vi "Skm To Dkm.vi"(8 "error in (no error)":errorcluster, 10 "error":i32, 11 "sKilo":string) -> (0 "error out":i32, 1 "function return":dbl, 2 "error out 2":errorcluster, 3 "sKilo out":string)   [LabVIEW 2023, in "POSCONV.lvlib"]
doc: "double SkmToDkm(char *sKilo, int *error);"
uses:
  POSCONV.lvlib
  C:/Users/J Gordon/Documents/Rail Tech/TV-HR/02 - Code/Modules/POSCONV/POSCONV.dll
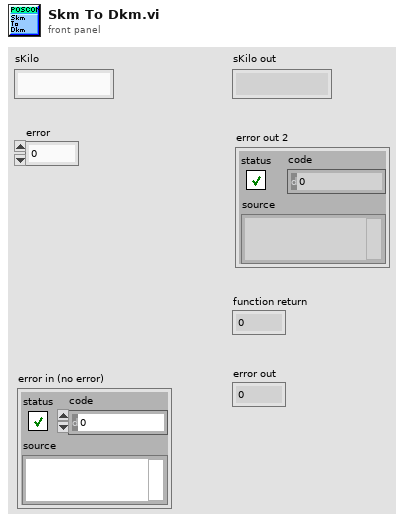
[diagram p1: front panel]
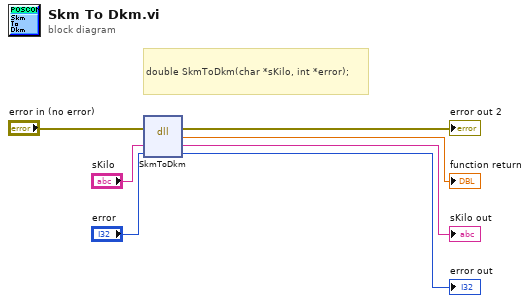
[diagram p0: block diagram]
diagram:
  # "double SkmToDkm(char *sKilo, int *error);"
  n1 = dll-call lib="C:/Users/J Gordon/Documents/Rail Tech/TV-HR/02 - Code/Modules/POSCONV/POSCONV.*" fn="SkmToDkm"(error in="error in (no error)", "sKilo"="sKilo", "error"="error") -> (error out=→"error out 2":errorcluster, →"function return":dbl, "sKilo"=→"sKilo out":string, "error"=→"error out":i32)  [unwired: 2 in, 1 out]
